vi "Main.vi"() -> ()   [LabVIEW 2022 SP3]
uses:
  <vilib>/Utility/error.llb/DialogType.ctl
panel:
  in  "File":T1(tab)
  out "out apc":string
  out "Торр":dbl format="%#_2g"
  out "Па":dbl format="%#_2e"
  out "мбар":dbl format="%#_2g"
  out "Торр":dbl(graph)
  out "AVARIA":bool
  in  "pyck ubp":bool
  in  "?":bool
  out "klapan":bool
  out "FORVAC":bool
  out "TYRBIK":bool
  in  "start otkachki":bool
  out "zatvor":bool
  out "stop apc":i32
  out "input voltage":i32
  out "output voltage":i32
  out "battary":i32
  out "Waveform Chart":dbl(graph)
  in  "DO":bool[](array[boolean])=[FALSE, FALSE, FALSE, FALSE] caption="Coils to Write"
  in  "DO 2":bool[](array[boolean])=[FALSE, FALSE, FALSE, FALSE] caption="Coils to Write"
  out "KONTROL2":bool
  out "kontrol1":bool
  in  "?":bool
  out "Zatvor":bool
  in  "Адрес ИБП":string="192.168.1.254"
  in  "Порт ИБП":u16=23
  in  "Адрес модуля DO":string="192.168.1.133"
  in  "Порт модуля DO":u16=502
  in  "Адрес модуля DO2":string="192.168.1.122"
  in  "Порт модуля DO2":u16=502
  in  "Давление менее":dbl=1.0
  in  "Давление менее":dbl=0.01
  out "reg 2":bool
  out "reg 1":bool
  # "Данные по источнику бесперебойного питания"
  # "Давление в вакуумной камере"
  # "Входное напряжение"
  # "В"
  # "Авария"
  # "Выходное напряжение"
  # "В"
  # "Клапан"
  # "Затвор"
  # "Заряд барареи"
  # "%"
  # "Выключение ИБП через"
  # "минут"
  # "Форвакуумный насос"
  # "Турбомолекулярный насос"
  # "Напряжение по вакумметру"
  # "В"
  # "Форвакуумный\n         насос"
  # "Турбомолекулярный\n            насос"
  # "Работа затвора"
  # "Контрольная точка 1"
  # "Контрольная точка 2"
  # "Затвор"
  # "Клапан"
  # "Давление менее 0,01 Торр"
  # "Давление менее 1 Торр"
  # "Контрольная точка 1"
  # "Контрольная точка 2"
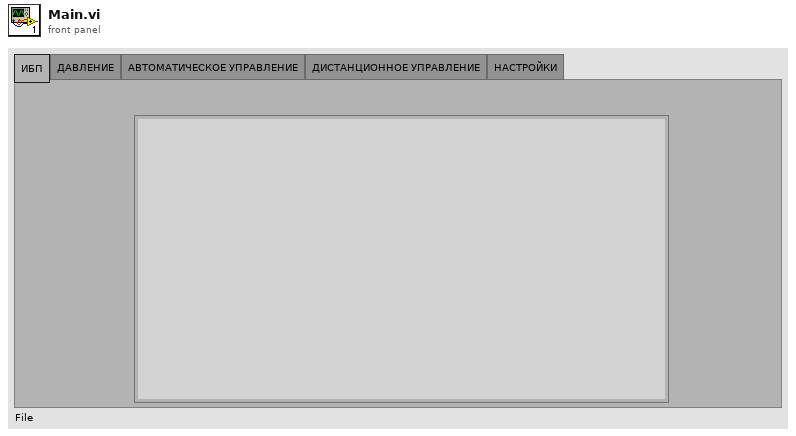
[diagram p1: front panel]
types:
  T1 = enum32{"ИБП", "ДАВЛЕНИЕ", "АВТОМАТИЧЕСКОЕ УПРАВЛЕНИЕ", "ДИСТАНЦИОННОЕ УПРАВЛЕНИЕ", "НАСТРОЙКИ"}
  T2 = enum16{"open", "replace", "create", "open or create", "replace or create", "replace or create with confirmation"}
  T3 = enum8{"Enabled", "Disabled", "Disabled and Grayed Out"}
  T4 = enum16{"Standard", "Buffered", "CRLF", "Immediate"}
  T5 = typedef "DialogType.ctl" = u16
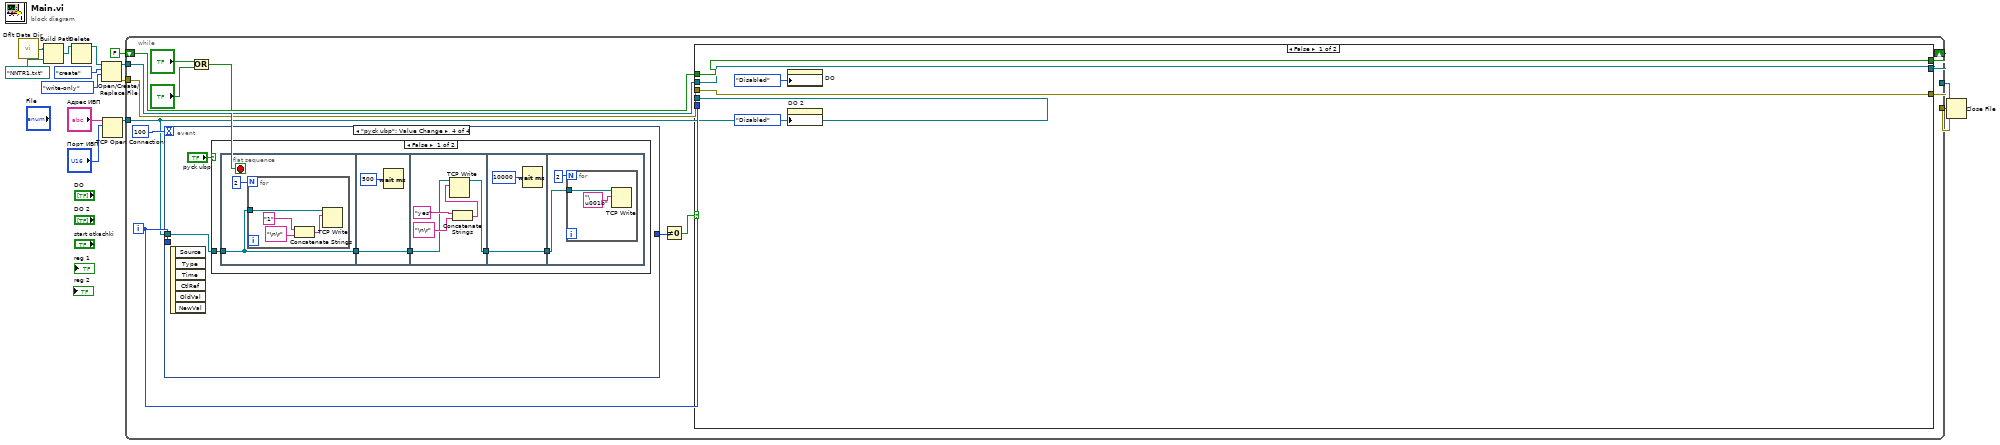
[diagram p0: block diagram]
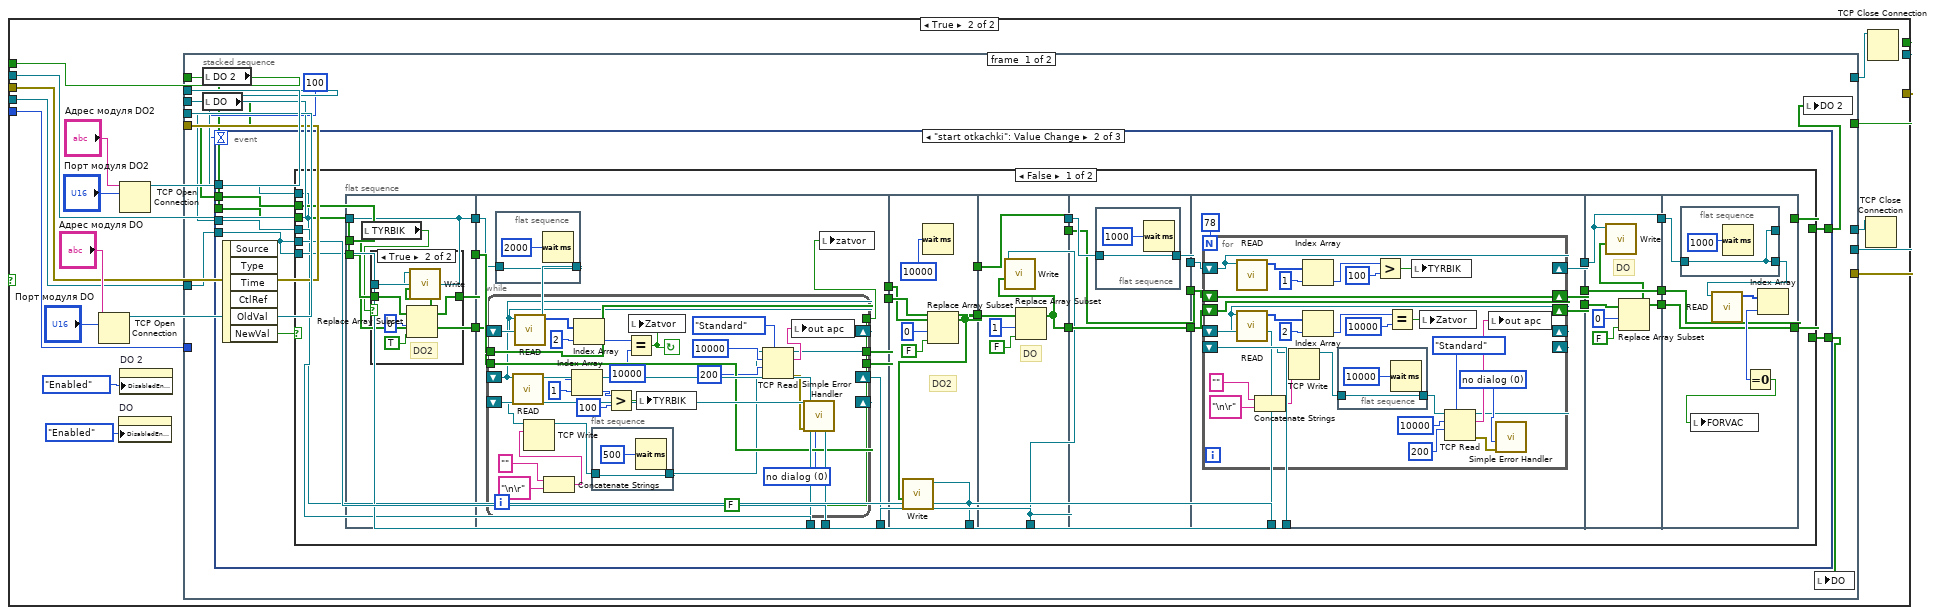
[diagram p2: hidden frame]
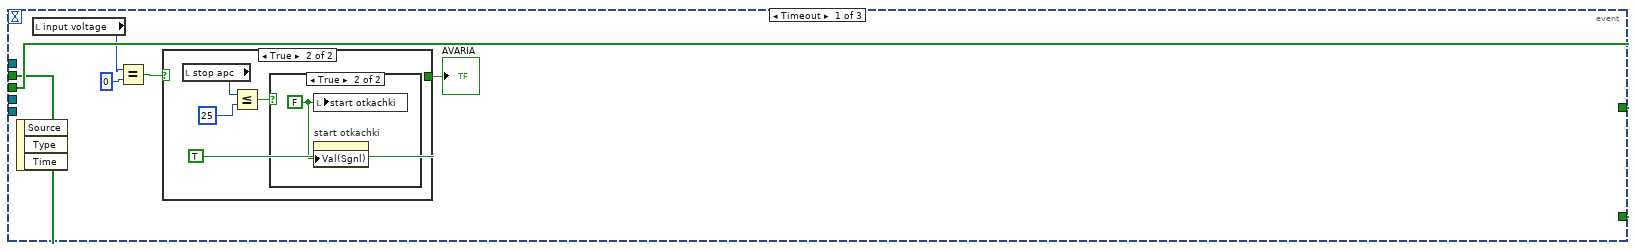
[diagram p3: hidden frame]
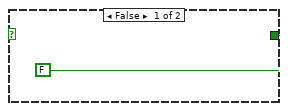
[diagram p4: hidden frame]
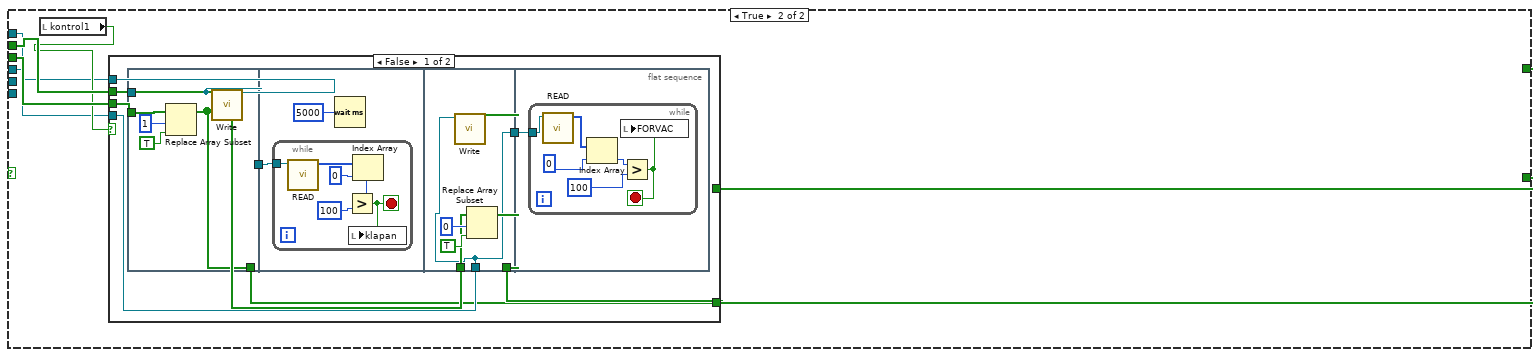
[diagram p7: hidden frame]
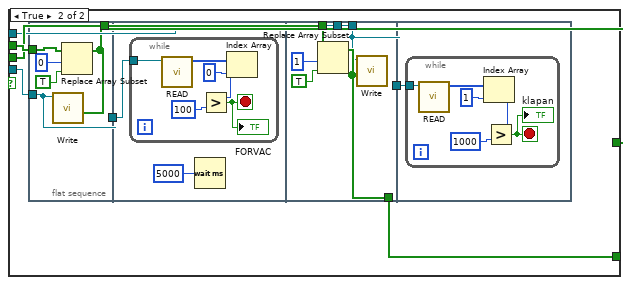
[diagram p8: hidden frame]
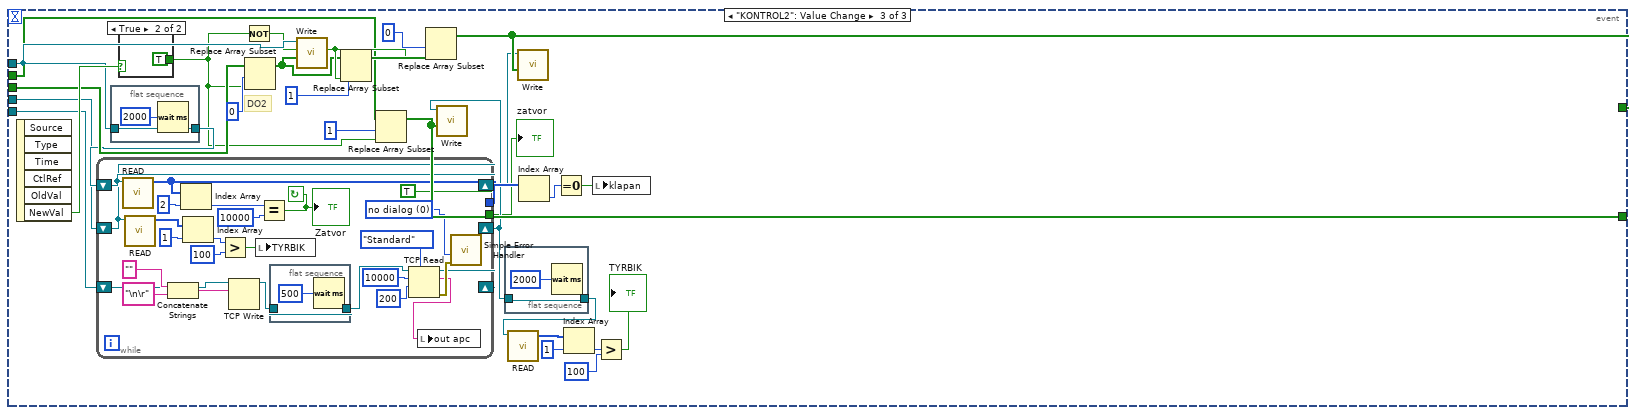
[diagram p9: hidden frame]
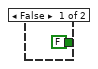
[diagram p10: hidden frame]
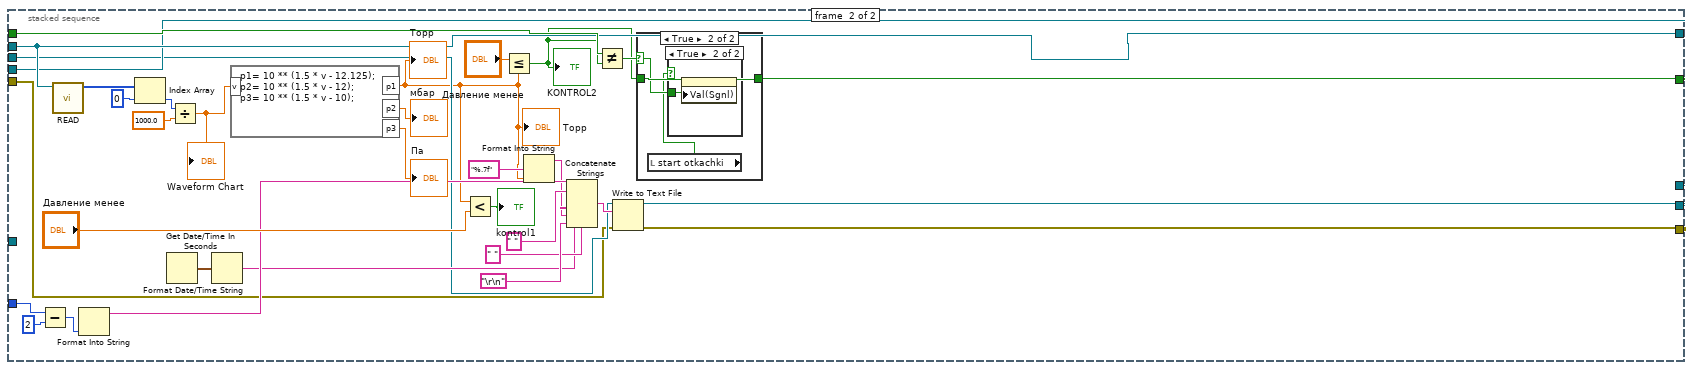
[diagram p11: hidden frame]
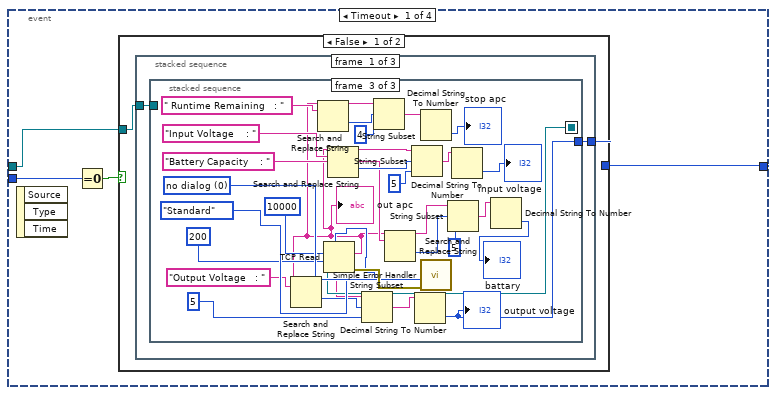
[diagram p14: hidden frame]
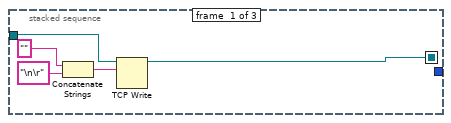
[diagram p15: hidden frame]
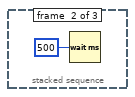
[diagram p16: hidden frame]
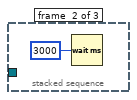
[diagram p17: hidden frame]
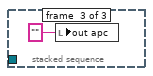
[diagram p18: hidden frame]
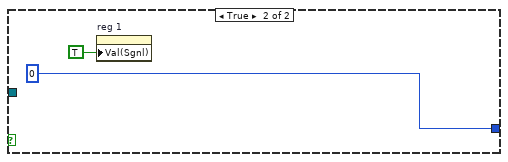
[diagram p19: hidden frame]
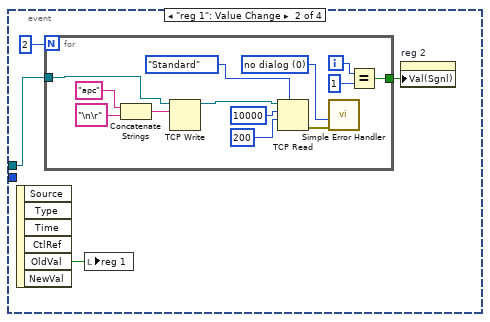
[diagram p20: hidden frame]
diagram:
  n1 = call <vilib>:"Dflt Data Dir.vi"() -> ("App:Default Data Directory"=w7:path)
  n2 = Build Path(base path=w7, name or relative path=path "NNTR1.txt" ("Path")) -> (appended path=w6:path)
  n3 = Delete(path (use dialog)=w6) -> (deleted path=w5:path)  [unwired: 4 in, 2 out]
  n4 = Open/Create/Replace File(file path (use dialog)=w5, operation (0:open)=T2."create", access (0:read/write)=enum16{"read/write", "read-only", "write-only"}."write-only") -> (refnum out=w2:refnum<file>, error out=w1:errorcluster)  [unwired: 3 in, 1 out]
  n5 = TCP Open Connection(address="Адрес ИБП", remote port or service name="Порт ИБП") -> (connection ID=w14:refnum<k5>)  [unwired: 3 in, 1 out]
  n6 = while {
    tunnel: w14 -> [w15]
    shift-right: [w24] -> _
    shift-left: FALSE -> [w25]
    tunnel: [w20] -> w10
    tunnel: [w19] -> w9
    tunnel: w2 -> [w18]
    tunnel: w1 -> [w17]
    i -> [w16]
    stop <- w23 stop-if-true
    n7 = event shown="[3] \"pyck ubp\": Value Change" {
      selector: _ -> [_ _ _ _]
      dyn-events: _ -> [_ _ _ _]
      timeout: 100 -> [_ _ _ _]
      tunnel: w15 -> [w410 w456 w473 w487]
      tunnel: w16 -> [w409 _ _ _]
      tunnel: [w407 _ _ _] -> w26
      event Timeout {
        n8 = event-data() -> ()  [unwired: 1 in, 3 out]
        n9 = Equal To 0?(x=w409) -> (x = 0?=w408:bool)
        n10 = case shown="False" w408 {
          tunnel: w410 -> [w412 _]
          tunnel: [w411 0] -> w407
          frame False {
            n11 = stacked-sequence {
              tunnel: w412 -> [w414 _ _]
              tunnel: [w413 _ _] -> w411
              frame #0 {
                n12 = stacked-sequence {
                  seq-local: [w419 _ _] -> [_ _ w446]
                  tunnel: w414 -> [w416 _ _]
                  tunnel: [_ _ w427] -> w413
                  frame #0 {
                    n13 = Concatenate Strings("" ("string"), "\n\r" ("string")) -> (w417:string)
                    n14 = TCP Write(connection ID=w416, data in=w417) -> (connection ID out=w419:refnum<k5>)  [unwired: 2 in, 2 out]
                  }
                  frame #1 {
                    n15 = Wait (ms)(milliseconds to wait=u32 500) -> ()  [unwired: 1 out]
                  }
                  frame #2 {
                    w450 = T5 0 items=["no dialog", "OK message", "continue or stop message", "OK message + warnings", "continue/stop + warnings"] ("type of dialog (OK msg:1)")
                    n16 = TCP Read(connection ID=w446, bytes to read=10000, 7:T4."Standard" ("mode (standard)"), 9:200 ("timeout ms (25000)")) -> (data out=w429:string, error out=w451:errorcluster)  [unwired: 1 in, 1 out]
                    "out apc" <- w429
                    n17 = Search and Replace String(input string=w429, search string="Output Voltage   : " ("search string/char (-)")) -> (result string=w432:string, offset past replacement=w431:i32)  [unwired: 6 in, 2 out]
                    n18 = Search and Replace String(input string=w429, search string=" Runtime Remaining   : " ("search string/char (-)")) -> (result string=w437:string, offset past replacement=w436:i32)  [unwired: 6 in, 2 out]
                    n19 = Search and Replace String(input string=w429, search string="Input Voltage    : " ("search string/char (-)")) -> (result string=w444:string, offset past replacement=w443:i32)  [unwired: 6 in, 2 out]
                    n20 = String Subset(string=w432, offset (0)=w431, length (rest)=5 ("length (rest)")) -> (substring=w428:string)
                    n21 = String Subset(string=w437, offset (0)=w436, length (rest)=4 ("length (rest)")) -> (substring=w426:string)
                    n22 = Search and Replace String(input string=w429, search string="Battery Capacity    : " ("search string/char (-)")) -> (result string=w440:string, offset past replacement=w439:i32)  [unwired: 6 in, 2 out]
                    n23 = String Subset(string=w444, offset (0)=w443, length (rest)=5 ("length (rest)")) -> (substring=w423:string)
                    n24 = Decimal String To Number(string=w428) -> (number=w427:i32)  [unwired: 2 in, 1 out]
                    "output voltage" <- w427
                    n25 = Decimal String To Number(string=w426) -> (number=→"stop apc":i32)  [unwired: 2 in, 1 out]
                    n26 = call <vilib>:"Simple Error Handler.vi"("type of dialog (OK msg:1)"=w450, "error in (no error)"=w451) -> ()  [unwired: 3 in, 5 out]
                    n27 = String Subset(string=w440, offset (0)=w439, length (rest)=5 ("length (rest)")) -> (substring=w421:string)
                    n28 = Decimal String To Number(string=w423) -> (number=→"input voltage":i32)  [unwired: 2 in, 1 out]
                    n29 = Decimal String To Number(string=w421) -> (number=→"battary":i32)  [unwired: 2 in, 1 out]
                  }
                }
              }
              frame #1 {
                n30 = Wait (ms)(milliseconds to wait=u32 3000) -> ()  [unwired: 1 out]
              }
              frame #2 {
                n31 = local write "out apc"("" ("data out 3")) -> ()
              }
            }
          }
          frame True {
            n32 = property on="reg 1" class="Bool (strict)"("Val(Sgnl)"=TRUE) -> ()  [unwired: 2 in, 2 out]
          }
        }
      }
      event "reg 1": Value Change {
        n33 = event-data() -> ("OldVal"=w458:bool)  [unwired: 1 in, 5 out]
        n34 = for {
          N: 2 -> [_]
          tunnel: [w461] -> w457
          tunnel: w456 -> [w460]
          i -> [w462]
          w470 = T5 0 items=["no dialog", "OK message", "continue or stop message", "OK message + warnings", "continue/stop + warnings"] ("type of dialog (OK msg:1)")
          n35 = Concatenate Strings("apc" ("string"), "\n\r" ("string")) -> (w465:string)
          n36 = TCP Write(connection ID=w460, data in=w465) -> (connection ID out=w471:refnum<k5>)  [unwired: 2 in, 2 out]
          n37 = TCP Read(connection ID=w471, bytes to read=10000, 7:T4."Standard" ("mode (standard)"), 9:200 ("timeout ms (25000)")) -> (error out=w472:errorcluster)  [unwired: 1 in, 2 out]
          n38 = call <vilib>:"Simple Error Handler.vi"("type of dialog (OK msg:1)"=w470, "error in (no error)"=w472) -> ()  [unwired: 3 in, 5 out]
          n39 = Equal?(x=w462, y=1) -> (x = y?=w461:bool)
        }
        n40 = local write "reg 1"(w458) -> ()
        n41 = property on="reg 2" class="Bool (strict)"("Val(Sgnl)"=w457) -> ()  [unwired: 2 in, 2 out]
      }
      event "reg 2": Value Change {
        n42 = event-data() -> ("OldVal"=w474:bool)  [unwired: 1 in, 5 out]
        n43 = local write "reg 2"(w474) -> ()
        n44 = for {
          N: 2 -> [_]
          tunnel: w473 -> [w476]
          w483 = T5 0 items=["no dialog", "OK message", "continue or stop message", "OK message + warnings", "continue/stop + warnings"] ("type of dialog (OK msg:1)")
          n45 = Concatenate Strings("1" ("string"), "\n\r" ("string")) -> (w478:string)
          n46 = TCP Write(connection ID=w476, data in=w478) -> (connection ID out=w484:refnum<k5>)  [unwired: 2 in, 2 out]
          n47 = TCP Read(connection ID=w484, bytes to read=10000, 7:T4."Standard" ("mode (standard)"), 9:200 ("timeout ms (25000)")) -> (error out=w485:errorcluster)  [unwired: 1 in, 2 out]
          n48 = call <vilib>:"Simple Error Handler.vi"("type of dialog (OK msg:1)"=w483, "error in (no error)"=w485) -> ()  [unwired: 3 in, 5 out]
        }
      }
      event "pyck ubp": Value Change {
        n49 = event-data() -> ()  [unwired: 1 in, 6 out]
        n50 = case shown="False" "pyck ubp" {
          tunnel: w487 -> [w490 w514]
          frame False {
            n51 = flat-sequence {
              tunnel: w490 -> [w494]
              tunnel: [w494] -> w492
              tunnel: w492 -> [w499]
              tunnel: [w499] -> w491
              tunnel: w491 -> [w502]
              tunnel: [w501] -> w489
              tunnel: w489 -> [w506]
              tunnel: [w506] -> w488
              tunnel: w488 -> [w509]
              frame #0 {
                n52 = for {
                  N: 2 -> [_]
                  tunnel: w494 -> [w495]
                  n53 = Concatenate Strings("1" ("string"), "\n\r" ("string")) -> (w497:string)
                  n54 = TCP Write(connection ID=w495, data in=w497) -> ()  [unwired: 2 in, 3 out]
                }
              }
              frame #1 {
                n55 = Wait (ms)(milliseconds to wait=u32 500) -> ()  [unwired: 1 out]
              }
              frame #2 {
                n56 = Concatenate Strings("yes" ("string"), "\n\r" ("string")) -> (w504:string)
                n57 = TCP Write(connection ID=w502, data in=w504) -> (connection ID out=w501:refnum<k5>)  [unwired: 2 in, 2 out]
              }
              frame #3 {
                n58 = Wait (ms)(milliseconds to wait=u32 10000) -> ()  [unwired: 1 out]
              }
              frame #4 {
                n59 = for {
                  N: 2 -> [_]
                  tunnel: w509 -> [w510]
                  n60 = TCP Write(connection ID=w510, data in="\u001b") -> ()  [unwired: 2 in, 3 out]
                }
              }
            }
          }
          frame True {
            n61 = flat-sequence {
              tunnel: w514 -> [w519]
              tunnel: [w518] -> w516
              tunnel: w516 -> [w525]
              tunnel: [w525] -> w515
              tunnel: w515 -> [w528]
              tunnel: [w527] -> w512
              tunnel: [w532] -> w513
              tunnel: w512 -> [w532]
              tunnel: w513 -> [w534]
              frame #0 {
                n62 = for {
                  N: 2 -> [_]
                  shift-right: [w520] -> w518
                  shift-left: w519 -> [w521]
                  n63 = Concatenate Strings("1" ("string"), "\n\r" ("string")) -> (w523:string)
                  n64 = TCP Write(connection ID=w521, data in=w523) -> (connection ID out=w520:refnum<k5>)  [unwired: 2 in, 2 out]
                }
              }
              frame #1 {
                n65 = Wait (ms)(milliseconds to wait=u32 500) -> ()  [unwired: 1 out]
              }
              frame #2 {
                n66 = Concatenate Strings("yes" ("string"), "\n\r" ("string")) -> (w530:string)
                n67 = TCP Write(connection ID=w528, data in=w530) -> (connection ID out=w527:refnum<k5>)  [unwired: 2 in, 2 out]
              }
              frame #3 {
                n68 = Wait (ms)(milliseconds to wait=u32 10000) -> ()  [unwired: 1 out]
              }
              frame #4 {
                n69 = for {
                  N: 2 -> [_]
                  tunnel: w534 -> [w537]
                  n70 = TCP Write(connection ID=w537, data in="\u001b") -> ()  [unwired: 2 in, 3 out]
                }
              }
            }
          }
        }
      }
    }
    n71 = Or(x="?", y="?") -> (x .or. y?=w23:bool)
    n72 = Not Equal To 0?(x=w26) -> (x != 0?=w27:bool)
    n73 = case shown="False" w27 {
      tunnel: [w31 w46] -> w24
      tunnel: w25 -> [w31 w45]
      tunnel: [w29 w39] -> w20
      tunnel: [w30 w38] -> w19
      tunnel: w18 -> [w29 w37]
      tunnel: w17 -> [w30 w36]
      tunnel: w16 -> [_ w35]
      tunnel: w15 -> [_ w34]
      frame False {
        n74 = property on="DO" class="Arr (strict)"("DisabledEnum"=T3."Disabled" ("Disabled")) -> ()  [unwired: 2 in, 2 out]
        n75 = property on="DO 2" class="Arr (strict)"("DisabledEnum"=T3."Disabled" ("Disabled")) -> ()  [unwired: 2 in, 2 out]
      }
      frame True {
        n76 = TCP Open Connection(address="Адрес модуля DO", remote port or service name="Порт модуля DO") -> (connection ID=w47:refnum<k5>)  [unwired: 3 in, 1 out]
        n77 = property on="DO" class="Arr (strict)"("DisabledEnum"=T3."Enabled" ("Disabled")) -> ()  [unwired: 2 in, 2 out]
        n78 = TCP Open Connection(address="Адрес модуля DO2", remote port or service name="Порт модуля DO2") -> (connection ID=w51:refnum<k5>)  [unwired: 3 in, 1 out]
        n79 = property on="DO 2" class="Arr (strict)"("DisabledEnum"=T3."Enabled" ("Disabled")) -> ()  [unwired: 2 in, 2 out]
        n80 = stacked-sequence {
          tunnel: w51 -> [w59 w391]
          tunnel: [_ w391] -> w50
          tunnel: w47 -> [w57 w390]
          tunnel: [_ w395] -> w46
          tunnel: w45 -> [_ w394]
          tunnel: [_ w390] -> w44
          tunnel: [_ w376] -> w39
          tunnel: [_ w375] -> w38
          tunnel: w37 -> [_ w374]
          tunnel: w36 -> [_ w373]
          tunnel: w35 -> [_ w371]
          tunnel: w34 -> [w52 _]
          frame #0 {
            n81 = local read "DO 2"() -> (w55:bool[])
            n82 = local read "DO"() -> (w56:bool[])
            n83 = event shown="[1] \"start otkachki\": Value Change" {
              selector: _ -> [_ _ _]
              dyn-events: _ -> [_ _ _]
              timeout: 100 -> [_ _ _]
              tunnel: w59 -> [_ w76 w329]
              tunnel: w57 -> [_ w77 w311]
              tunnel: w56 -> [w64 w78 w310]
              tunnel: w55 -> [w65 w75 w331]
              tunnel: [w64 w73 w332] -> w53
              tunnel: [w65 w74 w330] -> w54
              tunnel: w52 -> [_ w72 w308]
              event Timeout {
                n84 = event-data() -> ()  [unwired: 1 in, 3 out]
                n85 = local read "input voltage"() -> (w62:i32)
                n86 = Equal?(x=w62, y=0) -> (x = y?=w60:bool)
                n87 = case shown="True" w60 {
                  tunnel: [FALSE ("AVARIA") TRUE] -> w63
                  frame False {
                  }
                  frame True {
                    n88 = local read "stop apc"() -> (w68:i32)
                    n89 = Less Or Equal?(x=w68, y=25) -> (x <= y?=w67:bool)
                    n90 = case shown="True" w67 {
                      frame False {
                      }
                      frame True {
                        w71 = FALSE
                        n91 = local write "start otkachki"(w71) -> ()
                        n92 = property on="start otkachki" class="Bool (strict)"("Val(Sgnl)"=w71) -> ()  [unwired: 2 in, 2 out]
                      }
                    }
                  }
                }
                "AVARIA" <- w63
              }
              event "start otkachki": Value Change {
                n93 = event-data() -> ("NewVal"=w79:bool)  [unwired: 1 in, 5 out]
                n94 = case shown="False" w79 {
                  tunnel: w78 -> [w94 w239]
                  tunnel: w75 -> [w107 w238]
                  tunnel: w77 -> [w83 w233]
                  tunnel: w76 -> [w81 w236]
                  tunnel: [w97 w235] -> w74
                  tunnel: [w91 w234] -> w73
                  tunnel: w72 -> [w86 _]
                  tunnel: w72 -> [w85 _]
                  frame False {
                    n95 = flat-sequence {
                      tunnel: w107 -> [w112]
                      tunnel: w81 -> [w111]
                      tunnel: [w111] -> w106
                      tunnel: [w110] -> w102
                      tunnel: w94 -> [w109]
                      tunnel: [w109] -> w93
                      tunnel: w106 -> [w124]
                      tunnel: [w128] -> w103
                      tunnel: w102 -> [w127]
                      tunnel: [w126] -> w96
                      tunnel: w93 -> [w125]
                      tunnel: w86 -> [w122]
                      tunnel: w83 -> [w121]
                      tunnel: [w120] -> w84
                      tunnel: w103 -> [w163]
                      tunnel: w96 -> [w166]
                      tunnel: [w166] -> w95
                      tunnel: w81 -> [w162]
                      tunnel: [w161] -> w87
                      tunnel: w84 -> [w171]
                      tunnel: [w171] -> w105
                      tunnel: [w170] -> w98
                      tunnel: w95 -> [w169]
                      tunnel: [w168] -> w88
                      tunnel: w87 -> [w170]
                      tunnel: w105 -> [w177]
                      tunnel: [w176] -> w99
                      tunnel: w98 -> [w176]
                      tunnel: [w175] -> w89
                      tunnel: w88 -> [w175]
                      tunnel: [w174] -> w82
                      tunnel: [w183] -> w100
                      tunnel: w99 -> [w185]
                      tunnel: [w186] -> w90
                      tunnel: w89 -> [w187]
                      tunnel: w85 -> [w188]
                      tunnel: w82 -> [w182]
                      tunnel: w81 -> [w181]
                      tunnel: [w180] -> w80
                      tunnel: [w218] -> w104
                      tunnel: [w221] -> w101
                      tunnel: w100 -> [w221]
                      tunnel: [w220] -> w92
                      tunnel: w90 -> [w219]
                      tunnel: w80 -> [w218]
                      tunnel: w104 -> [w226]
                      tunnel: [w225] -> w97
                      tunnel: w101 -> [w225]
                      tunnel: [w224] -> w91
                      tunnel: w92 -> [w224]
                      frame #0 {
                        n96 = local read "TYRBIK"() -> (w108:bool)
                        n97 = case shown="True" w108 {
                          tunnel: w112 -> [w113 w118]
                          tunnel: w111 -> [_ w115]
                          tunnel: [w113 w114] -> w110
                          frame False {
                          }
                          frame True {
                            # "DO2"
                            n98 = Replace Array Subset(array=w118, new element=TRUE ("new element/subarray"), index=0) -> (w114:bool[])
                            n99 = call "Write.vi"("Discrete"=w114, "TCP Connection Refnum in"=w115) -> ()  [unwired: 10 in]
                          }
                        }
                      }
                      frame #1 {
                        n100 = while {
                          tunnel: [w156] -> w128
                          tunnel: w127 -> [w156]
                          tunnel: [w155] -> w126
                          tunnel: w125 -> [w155]
                          shift-right: [w151] -> _
                          shift-left: w123 -> [w151]
                          shift-right: [w144] -> _
                          shift-left: w122 -> [w138]
                          shift-right: [w132] -> w120
                          shift-left: w121 -> [w132]
                          tunnel: [FALSE] -> w119
                          stop <- w154 continue-if-true
                          w146 = T5 0 items=["no dialog", "OK message", "continue or stop message", "OK message + warnings", "continue/stop + warnings"] ("type of dialog (OK msg:1)")
                          n101 = call "READ.vi"("TCP Connection Refnum in"=w132) -> ("Registers"=w137:u16[])  [unwired: 10 in]
                          n102 = call "READ.vi"("TCP Connection Refnum in"=w151) -> ("Registers"=w157:u16[])  [unwired: 10 in]
                          n103 = Concatenate Strings("" ("string"), "\n\r" ("string")) -> (w142:string)
                          n104 = TCP Write(connection ID=w138, data in=w142) -> (connection ID out=w140:refnum<k5>)  [unwired: 2 in, 2 out]
                          n105 = Index Array(array=w137, index=1) -> (element=w136:u16)
                          n106 = Index Array(array=w157, index=2) -> (element=w153:u16)
                          n107 = flat-sequence {
                            tunnel: w140 -> [w159]
                            tunnel: [w159] -> w139
                            frame #0 {
                              n108 = Wait (ms)(milliseconds to wait=u32 500) -> ()  [unwired: 1 out]
                            }
                          }
                          n109 = Greater?(x=w136, y=u16 100) -> (0:w133:bool)
                          n110 = Equal?(x=w153, y=u16 10000) -> (x = y?=w154:bool)
                          n111 = local write "Zatvor"(w154) -> ()
                          n112 = local write "TYRBIK"(w133) -> ()
                          n113 = TCP Read(connection ID=w139, bytes to read=10000, 7:T4."Standard" ("mode (standard)"), 9:200 ("timeout ms (25000)")) -> (connection ID out=w144:refnum<k5>, data out=w150:string, error out=w145:errorcluster)  [unwired: 1 in]
                          n114 = local write "out apc"(w150) -> ()
                          n115 = call <vilib>:"Simple Error Handler.vi"("type of dialog (OK msg:1)"=w146, "error in (no error)"=w145) -> ()  [unwired: 3 in, 5 out]
                        }
                        n116 = flat-sequence {
                          tunnel: [w129] -> w123
                          tunnel: w124 -> [w129]
                          frame #0 {
                            n117 = Wait (ms)(milliseconds to wait=u32 2000) -> ()  [unwired: 1 out]
                          }
                        }
                        n118 = local write "zatvor"(w119) -> ()
                      }
                      frame #2 {
                        # "DO2"
                        n119 = Wait (ms)(milliseconds to wait=u32 10000) -> ()  [unwired: 1 out]
                        n120 = Replace Array Subset(array=w163, new element=FALSE ("new element/subarray"), index=0) -> (w161:bool[])
                        n121 = call "Write.vi"("Discrete"=w161, "TCP Connection Refnum in"=w162) -> ()  [unwired: 10 in]
                      }
                      frame #3 {
                        # "DO"
                        n122 = Replace Array Subset(array=w169, new element=FALSE ("new element/subarray"), index=1) -> (w168:bool[])
                        n123 = call "Write.vi"("Discrete"=w168, "TCP Connection Refnum in"=w171) -> ()  [unwired: 10 in]
                      }
                      frame #4 {
                        n124 = flat-sequence {
                          tunnel: [w178] -> w174
                          tunnel: w177 -> [w178]
                          frame #0 {
                            n125 = Wait (ms)(milliseconds to wait=u32 1000) -> ()  [unwired: 1 out]
                          }
                        }
                      }
                      frame #5 {
                        n126 = for {
                          N: 78 -> [_]
                          shift-right: [w209] -> _
                          shift-left: w188 -> [w202]
                          shift-right: [w208] -> w186
                          shift-left: w187 -> [w208]
                          shift-right: [w207] -> w183
                          shift-left: w185 -> [w207]
                          shift-right: [w189] -> _
                          shift-left: w181 -> [w189]
                          shift-right: [w190] -> w180
                          shift-left: w182 -> [w190]
                          w211 = T5 0 items=["no dialog", "OK message", "continue or stop message", "OK message + warnings", "continue/stop + warnings"] ("type of dialog (OK msg:1)")
                          n127 = call "READ.vi"("TCP Connection Refnum in"=w190) -> ("Registers"=w195:u16[])  [unwired: 10 in]
                          n128 = call "READ.vi"("TCP Connection Refnum in"=w189) -> ("Registers"=w199:u16[])  [unwired: 10 in]
                          n129 = Concatenate Strings("" ("string"), "\n\r" ("string")) -> (w204:string)
                          n130 = TCP Write(connection ID=w202, data in=w204) -> (connection ID out=w206:refnum<k5>)  [unwired: 2 in, 2 out]
                          n131 = Index Array(array=w195, index=1) -> (element=w194:u16)
                          n132 = Index Array(array=w199, index=2) -> (element=w197:u16)
                          n133 = flat-sequence {
                            tunnel: w206 -> [w216]
                            tunnel: [w216] -> w201
                            frame #0 {
                              n134 = Wait (ms)(milliseconds to wait=u32 10000) -> ()  [unwired: 1 out]
                            }
                          }
                          n135 = Greater?(x=w194, y=u16 100) -> (0:w191:bool)
                          n136 = Equal?(x=w197, y=u16 10000) -> (x = y?=w198:bool)
                          n137 = local write "TYRBIK"(w191) -> ()
                          n138 = local write "Zatvor"(w198) -> ()
                          n139 = TCP Read(connection ID=w201, bytes to read=10000, 7:T4."Standard" ("mode (standard)"), 9:200 ("timeout ms (25000)")) -> (connection ID out=w209:refnum<k5>, data out=w215:string, error out=w210:errorcluster)  [unwired: 1 in]
                          n140 = local write "out apc"(w215) -> ()
                          n141 = call <vilib>:"Simple Error Handler.vi"("type of dialog (OK msg:1)"=w211, "error in (no error)"=w210) -> ()  [unwired: 3 in, 5 out]
                        }
                      }
                      frame #6 {
                        # "DO"
                        n142 = Replace Array Subset(array=w219, new element=FALSE ("new element/subarray"), index=0) -> (w220:bool[])
                        n143 = call "Write.vi"("Discrete"=w220, "TCP Connection Refnum in"=w218) -> ()  [unwired: 10 in]
                      }
                      frame #7 {
                        n144 = flat-sequence {
                          tunnel: w226 -> [w231]
                          tunnel: [w231] -> w230
                          tunnel: [w231] -> _
                          frame #0 {
                            n145 = Wait (ms)(milliseconds to wait=u32 1000) -> ()  [unwired: 1 out]
                          }
                        }
                        n146 = call "READ.vi"("TCP Connection Refnum in"=w230) -> ("Registers"=w229:u16[])  [unwired: 10 in]
                        n147 = Index Array(array=w229) -> (element=w228:u16)  [unwired: 1 in]
                        n148 = Equal To 0?(x=w228) -> (x = 0?=w227:bool)
                        n149 = local write "FORVAC"(w227) -> ()
                      }
                    }
                  }
                  frame True {
                    n150 = local read "kontrol1"() -> (w237:bool)
                    n151 = case shown="False" w237 {
                      tunnel: w239 -> [w247 w280]
                      tunnel: w238 -> [w245 w279]
                      tunnel: w236 -> [w244 w275]
                      tunnel: [w240 w277] -> w235
                      tunnel: [w246 w276] -> w234
                      tunnel: w233 -> [w243 w273]
                      frame False {
                        n152 = flat-sequence {
                          tunnel: w245 -> [w250]
                          tunnel: w244 -> [w249]
                          tunnel: [w249] -> w241
                          tunnel: [w248] -> w240
                          tunnel: w241 -> [w253]
                          tunnel: w247 -> [w263]
                          tunnel: [w262] -> w246
                          tunnel: w243 -> [w261]
                          tunnel: [w261] -> w242
                          tunnel: w242 -> [w266]
                          frame #0 {
                            n153 = Replace Array Subset(array=w250, new element=TRUE ("new element/subarray"), index=1) -> (w248:bool[])
                            n154 = call "Write.vi"("Discrete"=w248, "TCP Connection Refnum in"=w249) -> ()  [unwired: 10 in]
                          }
                          frame #1 {
                            n155 = while {
                              tunnel: w253 -> [w255]
                              stop <- w256 stop-if-true
                              n156 = call "READ.vi"("TCP Connection Refnum in"=w255) -> ("Registers"=w259:u16[])  [unwired: 10 in]
                              n157 = Index Array(array=w259, index=0) -> (element=w257:u16)
                              n158 = Greater?(x=w257, y=u16 100) -> (0:w256:bool)
                              n159 = local write "klapan"(w256) -> ()
                            }
                            n160 = Wait (ms)(milliseconds to wait=u32 5000) -> ()  [unwired: 1 out]
                          }
                          frame #2 {
                            n161 = Replace Array Subset(array=w263, new element=TRUE ("new element/subarray"), index=0) -> (w262:bool[])
                            n162 = call "Write.vi"("Discrete"=w262, "TCP Connection Refnum in"=w261) -> ()  [unwired: 10 in]
                          }
                          frame #3 {
                            n163 = while {
                              tunnel: w266 -> [w267]
                              stop <- w268 stop-if-true
                              n164 = call "READ.vi"("TCP Connection Refnum in"=w267) -> ("Registers"=w271:u16[])  [unwired: 10 in]
                              n165 = Index Array(array=w271, index=0) -> (element=w269:u16)
                              n166 = Greater?(x=w269, y=u16 100) -> (0:w268:bool)
                              n167 = local write "FORVAC"(w268) -> ()
                            }
                          }
                        }
                      }
                      frame True {
                        n168 = flat-sequence {
                          tunnel: w280 -> [w283]
                          tunnel: w273 -> [w282]
                          tunnel: [w282] -> w278
                          tunnel: [w281] -> w276
                          tunnel: w278 -> [w287]
                          tunnel: w279 -> [w296]
                          tunnel: w275 -> [w294]
                          tunnel: [w295] -> w277
                          tunnel: w275 -> [_]
                          tunnel: [w294] -> w274
                          tunnel: w274 -> [w299]
                          frame #0 {
                            n169 = Replace Array Subset(array=w283, new element=TRUE ("new element/subarray"), index=0) -> (w281:bool[])
                            n170 = call "Write.vi"("Discrete"=w281, "TCP Connection Refnum in"=w282) -> ()  [unwired: 10 in]
                          }
                          frame #1 {
                            n171 = while {
                              tunnel: w287 -> [w288]
                              stop <- w289 stop-if-true
                              n172 = call "READ.vi"("TCP Connection Refnum in"=w288) -> ("Registers"=w292:u16[])  [unwired: 10 in]
                              n173 = Index Array(array=w292, index=0) -> (element=w290:u16)
                              n174 = Greater?(x=w290, y=u16 100) -> (0:w289:bool)
                              "FORVAC" <- w289
                            }
                            n175 = Wait (ms)(milliseconds to wait=u32 5000) -> ()  [unwired: 1 out]
                          }
                          frame #2 {
                            n176 = Replace Array Subset(array=w296, new element=TRUE ("new element/subarray"), index=1) -> (w295:bool[])
                            n177 = call "Write.vi"("Discrete"=w295, "TCP Connection Refnum in"=w294) -> ()  [unwired: 10 in]
                          }
                          frame #3 {
                            n178 = while {
                              tunnel: w299 -> [w300]
                              stop <- w301 stop-if-true
                              n179 = call "READ.vi"("TCP Connection Refnum in"=w300) -> ("Registers"=w302:u16[])  [unwired: 10 in]
                              n180 = Index Array(array=w302, index=1) -> (element=w305:u16)
                              n181 = Greater?(x=w305, y=u16 1000) -> (0:w301:bool)
                              "klapan" <- w301
                            }
                          }
                        }
                      }
                    }
                  }
                }
              }
              event "KONTROL2": Value Change {
                # "DO2"
                n182 = event-data() -> ("NewVal"=w333:bool)  [unwired: 1 in, 5 out]
                n183 = while {
                  tunnel: [w358] -> w316
                  shift-right: [w357] -> w312
                  shift-left: w313 -> [w357]
                  shift-right: [w345] -> w309
                  shift-left: w311 -> [w345]
                  shift-right: [w344] -> _
                  shift-left: w308 -> [w339]
                  tunnel: [TRUE] -> w306
                  stop <- w359 continue-if-true
                  w355 = T5 0 items=["no dialog", "OK message", "continue or stop message", "OK message + warnings", "continue/stop + warnings"] ("type of dialog (OK msg:1)")
                  n184 = call "READ.vi"("TCP Connection Refnum in"=w357) -> ("Registers"=w358:u16[])  [unwired: 10 in]
                  n185 = call "READ.vi"("TCP Connection Refnum in"=w345) -> ("Registers"=w350:u16[])  [unwired: 10 in]
                  n186 = Concatenate Strings("" ("string"), "\n\r" ("string")) -> (w342:string)
                  n187 = Index Array(array=w358, index=2) -> (element=w361:u16)
                  n188 = Index Array(array=w350, index=1) -> (element=w349:u16)
                  n189 = Greater?(x=w349, y=u16 100) -> (0:w346:bool)
                  n190 = TCP Write(connection ID=w339, data in=w342) -> (connection ID out=w340:refnum<k5>)  [unwired: 2 in, 2 out]
                  n191 = local write "TYRBIK"(w346) -> ()
                  n192 = Equal?(x=w361, y=u16 10000) -> (x = y?=w359:bool)
                  "Zatvor" <- w359
                  n193 = flat-sequence {
                    tunnel: w340 -> [w363]
                    tunnel: [w363] -> w338
                    frame #0 {
                      n194 = Wait (ms)(milliseconds to wait=u32 500) -> ()  [unwired: 1 out]
                    }
                  }
                  n195 = TCP Read(connection ID=w338, bytes to read=10000, 7:T4."Standard" ("mode (standard)"), 9:200 ("timeout ms (25000)")) -> (connection ID out=w344:refnum<k5>, data out=w351:string, error out=w356:errorcluster)  [unwired: 1 in]
                  n196 = local write "out apc"(w351) -> ()
                  n197 = call <vilib>:"Simple Error Handler.vi"("type of dialog (OK msg:1)"=w355, "error in (no error)"=w356) -> ()  [unwired: 3 in, 5 out]
                }
                "zatvor" <- w306
                n198 = flat-sequence {
                  tunnel: [w335] -> w313
                  tunnel: w329 -> [w335]
                  frame #0 {
                    n199 = Wait (ms)(milliseconds to wait=u32 2000) -> ()  [unwired: 1 out]
                  }
                }
                n200 = case shown="True" w333 {
                  tunnel: [FALSE TRUE] -> w307
                  frame False {
                  }
                  frame True {
                  }
                }
                n201 = Not(x=w307) -> (.not. x?=w318:bool)
                n202 = Replace Array Subset(array=w331, new element=w307, index=0) -> (w317:bool[])
                n203 = call "Write.vi"("Discrete"=w317, "TCP Connection Refnum in"=w329) -> ()  [unwired: 10 in]
                n204 = Replace Array Subset(array=w317, new element=w318, index=1) -> (w319:bool[])
                n205 = Replace Array Subset(array=w310, new element=w307, index=1) -> (w332:bool[])
                n206 = Replace Array Subset(array=w319, new element=w318, index=0) -> (w330:bool[])
                n207 = call "Write.vi"("Discrete"=w332, "TCP Connection Refnum in"=w309) -> ()  [unwired: 10 in]
                n208 = flat-sequence {
                  tunnel: [w365] -> w327
                  tunnel: w309 -> [w365]
                  frame #0 {
                    n209 = Wait (ms)(milliseconds to wait=u32 2000) -> ()  [unwired: 1 out]
                  }
                }
                n210 = call "READ.vi"("TCP Connection Refnum in"=w327) -> ("Registers"=w326:u16[])  [unwired: 10 in]
                n211 = call "Write.vi"("Discrete"=w330, "TCP Connection Refnum in"=w312) -> ()  [unwired: 10 in]
                n212 = Index Array(array=w316) -> (element=w315:u16)  [unwired: 1 in]
                n213 = Equal To 0?(x=w315) -> (x = 0?=w314:bool)
                n214 = Index Array(array=w326, index=1) -> (element=w325:u16)
                n215 = local write "klapan"(w314) -> ()
                n216 = Greater?(x=w325, y=u16 100) -> (0:→"TYRBIK":bool)
              }
            }
            n217 = local write "DO 2"(w54) -> ()
            n218 = local write "DO"(w53) -> ()
          }
          frame #1 {
            n219 = Subtract(x=w371, y=2) -> (x-y=w369:i32)
            n220 = call "READ.vi"("TCP Connection Refnum in"=w391) -> ("Registers"=w392:u16[])  [unwired: 10 in]
            n221 = Format Into String(w369) -> (resulting string=w380:string)  [unwired: 3 in, 1 out]
            n222 = Index Array(array=w392, index=0) -> (element=w399:u16)
            n223 = Get Date/Time In Seconds() -> (seconds since 1Jan1904=w379:timestamp)
            n224 = Divide(x=w399, y=1000.0) -> (x/y=w398:dbl)
            "Waveform Chart" <- w398
            n225 = Format Date/Time String(seconds (now)=w379) -> (date/time string=w377:string)  [unwired: 2 in]
            n226 = formula code="p1= 10 ** (1.5 * v - 12.125);\np2= 10 ** (1.5 * v - 12);\np3= 10 ** (1.5 * v - 10);"("v"=w398) -> ("p1"=w372:dbl, "p2"=→"мбар":dbl, "p3"=→"Па":dbl)
            "Торр" <- w372
            "Торр" <- w372
            n227 = Less?(x=w372, y="Давление менее") -> (x < y?=→"kontrol1":bool)
            n228 = Less Or Equal?(x=w372, y="Давление менее") -> (x <= y?=w389:bool)
            "KONTROL2" <- w389
            n229 = Format Into String(format string="%.7f", w372) -> (resulting string=w378:string)  [unwired: 2 in, 1 out]
            n230 = Concatenate Strings(w380, " " ("string"), w377, " " ("string"), w378, "\r\n") -> (w381:string)
            n231 = Not Equal?(x=w394, y=w389) -> (x != y?=w393:bool)
            n232 = Write to Text File(file (use dialog)=w374, text=w381, error in=w373) -> (refnum out=w376:refnum<file>, error out=w375:errorcluster)  [unwired: 1 in, 1 out]
            n233 = case shown="True" w393 {
              selector: w393 -> [_ w404]
              tunnel: [w402 w405] -> w395
              tunnel: w389 -> [w402 w405]
              frame False {
              }
              frame True {
                n234 = local read "start otkachki"() -> (w403:bool)
                n235 = case shown="True" w403 {
                  tunnel: w404 -> [_ w406]
                  frame False {
                  }
                  frame True {
                    n236 = property on="KONTROL2" class="Bool (strict)"("Val(Sgnl)"=w406) -> ()  [unwired: 2 in, 2 out]
                  }
                }
              }
            }
          }
        }
        n237 = TCP Close Connection(connection ID=w44) -> ()  [unwired: 2 in, 2 out]
        n238 = TCP Close Connection(connection ID=w50) -> ()  [unwired: 2 in, 2 out]
      }
    }
  }
  n239 = Close File(refnum=w10, error in=w9) -> ()  [unwired: 2 out]
